vi "DAQmxAcq INIT.vi"(7 "physical channels":tag="Dev2/ai0", 8 "error in":errorcluster, 11 "DAQmxChannel":T1) -> (0 "error out":errorcluster, 3 "task out":refnum<k21>)   [LabVIEW 2020]
uses:
  <vilib>/DAQmx/create/channels.llb/DAQmx Create Channel (AI-Voltage-Basic).vi
  <vilib>/DAQmx/configure/timing.llb/DAQmx Timing (Sample Clock).vi
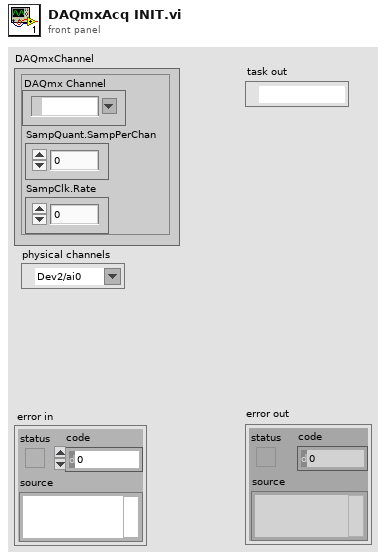
[diagram p1: front panel]
types:
  T1 = cluster{"SampClk.Rate":dbl, "SampQuant.SampPerChan":i32, "DAQmx Channel":refnum<k21>}
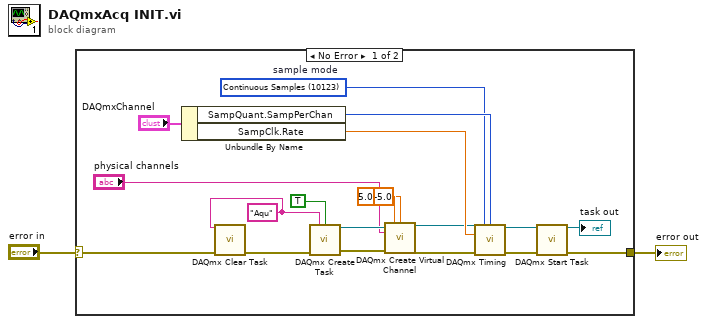
[diagram p0: block diagram]
diagram:
  n1 = case shown="No Error" "error in" {
    selector: "error in" -> [w5 w22]
    tunnel: [w17 w22] -> w2
    frame No Error {
      w6 = "Aqu" ("task name")
      w19 = 10123 items=["Finite Samples"=10178, "Continuous Samples"=10123, "Hardware Timed Single Point"=12522]  # sample mode
      n2 = Unbundle By Name("DAQmxChannel") -> ("SampQuant.SampPerChan"=w21:i32, "SampClk.Rate"=w20:dbl)
      n3 = call <vilib>:"DAQmx Clear Task.vi"("task in"=w6, "error in"=w5) -> ("error out"=w7:errorcluster)  [unwired: 13 in]
      n4 = call <vilib>:"DAQmx Create Task.vi"("new task name"=w6, "auto cleanup"=TRUE, "error in"=w7) -> ("task out"=w13:refnum<k21>, "error out"=w10:errorcluster)  [unwired: 11 in]
      n5 = call-poly <vilib>:"DAQmx Create Virtual Channel.vi"("task in"=w13, "maximum value"=5.0, "minimum value"=-5.0, "physical channels"="physical channels", "error in"=w10) -> ("task out"=w12:refnum<k21>, "error out"=w11:errorcluster)  [unwired: 9 in]
      n6 = call-poly <vilib>:"DAQmx Timing.vi"("task/channels in"=w12, "sample mode"=w19, "samples per channel"=w21, "rate"=w20, "error in"=w11) -> ("task out"=w16:refnum<k21>, "error out"=w18:errorcluster)  [unwired: 9 in]
      n7 = call <vilib>:"DAQmx Start Task.vi"("task/channels in"=w16, "error in"=w18) -> ("task out"=→"task out":refnum<k21>, "error out"=w17:errorcluster)  [unwired: 12 in]
    }
    frame Error {
    }
  }
  "error out" <- w2
